vi "andor camera info.vi"(2 "error in":errorcluster) -> (0 "error out":errorcluster, 1 "Andor Camera Properties":T1)   [LabVIEW 2015]
uses:
  andor camera properties.ctl
  Program Files (x86)/BDS2006/ATMCD32D.DLL
panel:
  out "VS Speeds (us/row)":sgl[](array[numeric])
  out "Number of VS Speeds":i32
  out "Preamp Gain Settings":sgl[](array[numeric])
  out "Number of Preamp Gains":i32
  out "Pixel V (um)":sgl
  out "Pixel H (um)":sgl
  out "Pixel Frequencies (MHz)\n(for each channel)":sgl[][](array[numeric])
  out "Number of HS Speeds\n(for each Channel)":i32[](array[numeric])
  out "Number of AD Channels":i32
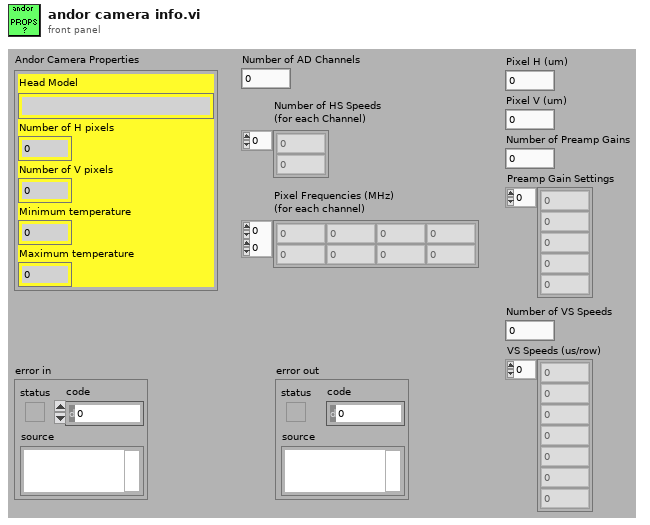
[diagram p1: front panel]
types:
  T1 = typedef "andor camera properties.ctl" = cluster{"Head Model":string, "Number of H pixels":i32, "Number of V pixels":i32, "Minimum temperature":i32, "Maximum temperature":i32}
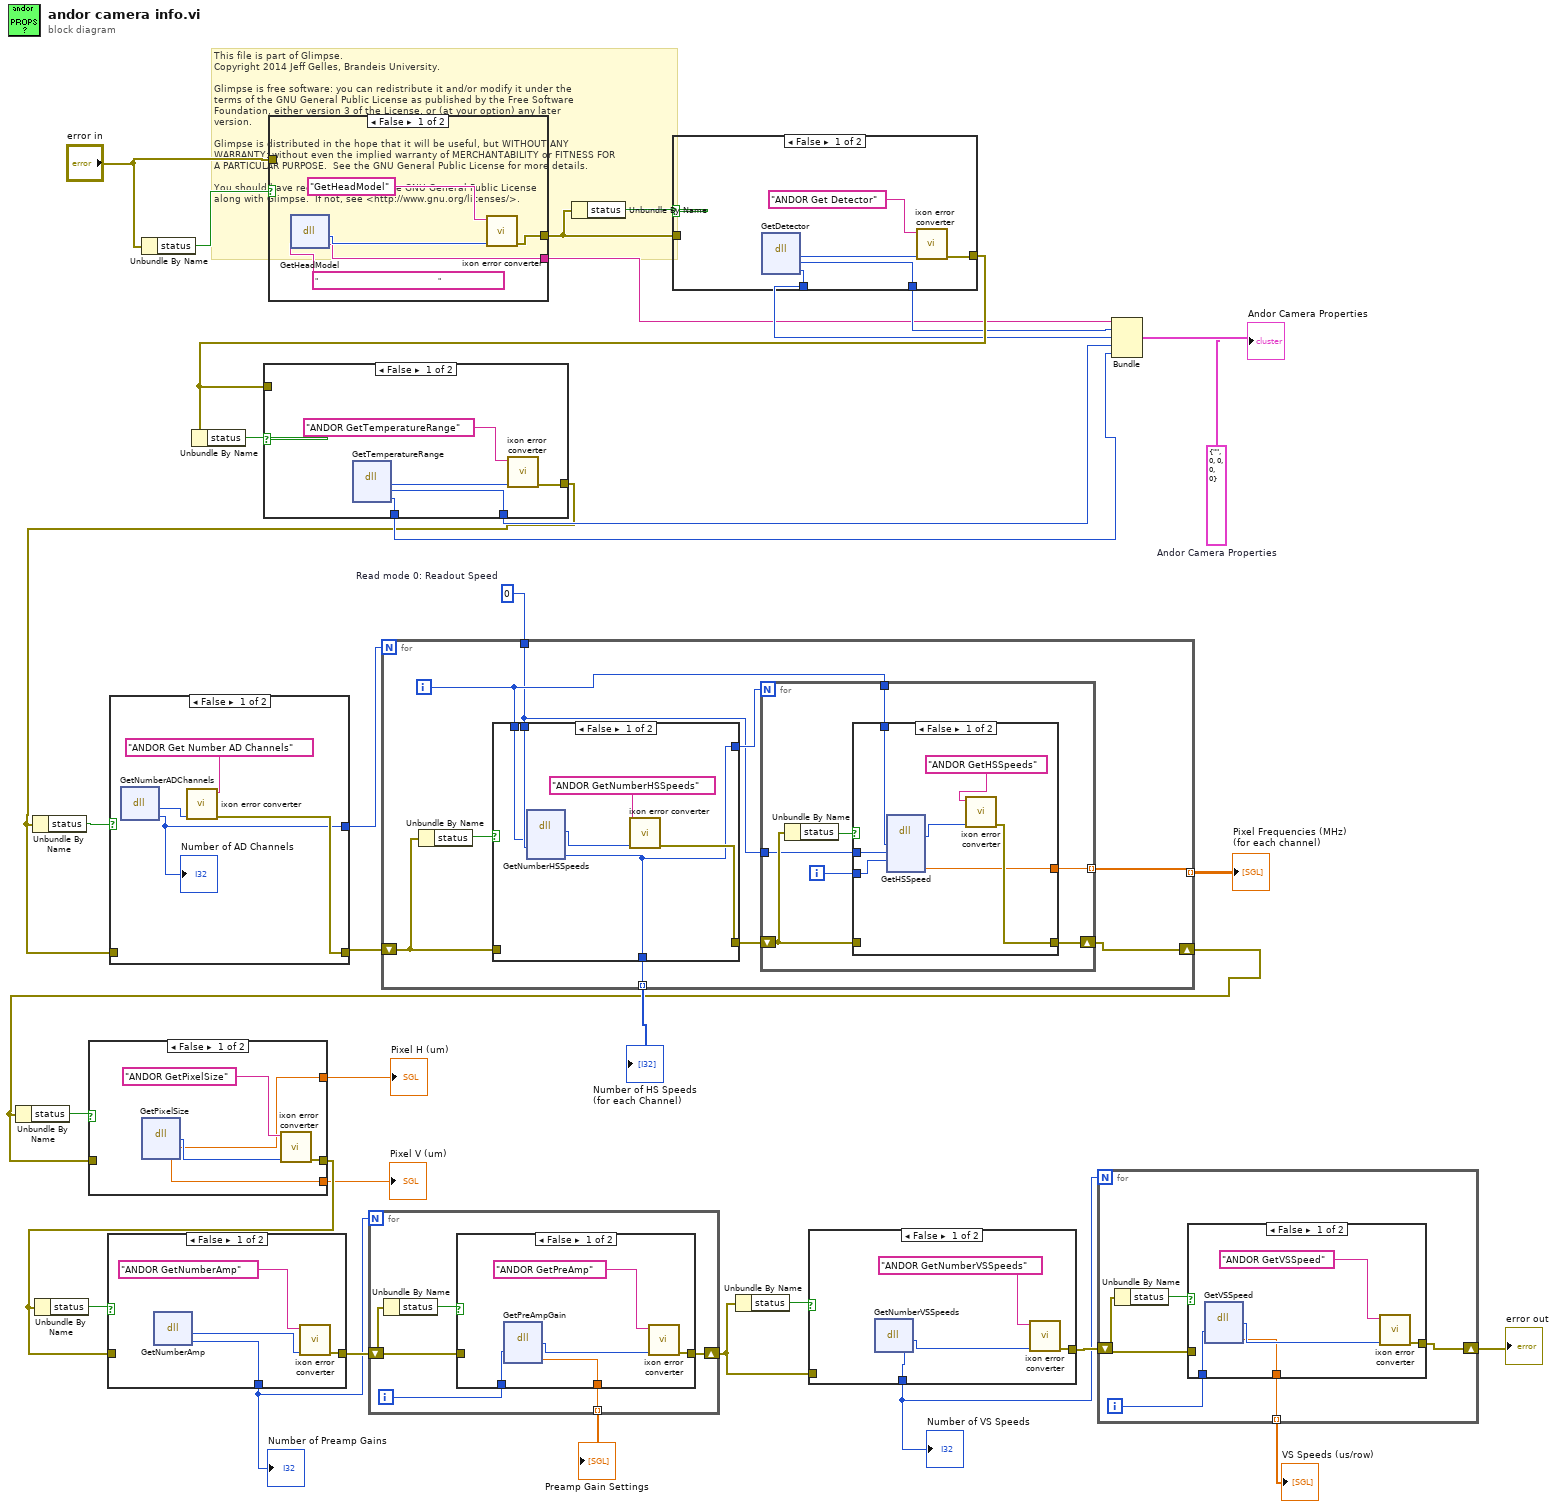
[diagram p0: block diagram]
diagram:
  w19 = 0  # Read mode 0: Readout Speed
  w27 = T1 {"Head Model"="", "Number of H pixels"=0, "Number of V pixels"=0, "Minimum temperature"=0, "Maximum temperature"=0}  # Andor Camera Properties
  # "This file is part of Glimpse. \nCopyright 2014 Jeff Gelles, Brandeis University.    \n\nGlimpse is free software: you can redistribute it and/or modify it under the \nterms of the GNU General Public License as published by the Free Software \nFoundation, either version 3 of the License, or (at your option) any later \nversion.\n\nGlimpse is distributed in the hope that it will be useful, but WITHOUT ANY \nWARRANTY; without even the implied warranty of MERCHANTABILITY or FITNESS FOR \nA PARTICULAR PURPOSE.  See the GNU General Public License for more details.\n\nYou should have received a copy of the GNU General Public License\nalong with Glimpse.  If not, see <http://www.gnu.org/licenses/>."
  n1 = Unbundle By Name("error in") -> ("status"=w24:bool)
  n2 = case shown="False" w24 {
    tunnel: [w38 w41] -> w26
    tunnel: "error in" -> [_ w41]
    tunnel: [w36 _] -> w28
    frame False {
      n3 = dll-call lib="C:/Program Files (x86)/BDS2006/Atmcd32d.dll" fn="GetHeadModel"("                                                            ") -> (w40:u32, w36:string)  [unwired: 3 in, 2 out]
      n4 = call "ixon error converter.vi"("Andor error code"=w40, "source"="GetHeadModel") -> ("error out"=w38:errorcluster)  [unwired: 5 out]
    }
    frame True {
    }
  }
  n5 = Unbundle By Name(w26) -> ("status"=w23:bool)
  n6 = case shown="False" w23 {
    tunnel: [w45 w47] -> w33
    tunnel: w26 -> [_ w47]
    tunnel: [w43 _] -> w29
    tunnel: [w42 _] -> w30
    frame False {
      n7 = dll-call lib="C:/Program Files (x86)/BDS2006/Atmcd32d.dll" fn="GetDetector" label="Get Detector"() -> (w44:u32, w42:i32, w43:i32)  [unwired: 3 in, 4 out]
      n8 = call "ixon error converter.vi"("Andor error code"=w44, "source"="ANDOR Get Detector") -> ("error out"=w45:errorcluster)  [unwired: 5 out]
    }
    frame True {
    }
  }
  n9 = Unbundle By Name(w33) -> ("status"=w32:bool)
  n10 = case shown="False" w32 {
    tunnel: [w51 w53] -> w22
    tunnel: [w49 _] -> w35
    tunnel: [w48 _] -> w34
    tunnel: w33 -> [_ w53]
    frame False {
      n11 = dll-call lib="C:/Program Files (x86)/BDS2006/Atmcd32d.dll" fn="GetTemperatureRange"() -> (w50:u32, w48:i32, w49:i32)  [unwired: 3 in, 4 out]
      n12 = call "ixon error converter.vi"("Andor error code"=w50, "source"="ANDOR GetTemperatureRange") -> ("error out"=w51:errorcluster)  [unwired: 5 out]
    }
    frame True {
    }
  }
  n13 = Unbundle By Name(w22) -> ("status"=w21:bool)
  n14 = case shown="False" w21 {
    tunnel: [w55 w58] -> w20
    tunnel: w22 -> [_ w58]
    tunnel: [w54 _] -> w1
    frame False {
      n15 = dll-call lib="C:/Program Files (x86)/BDS2006/Atmcd32d.dll" fn="GetNumberADChannels" label="Get Number AD Channels"() -> (w56:u32, w54:i32)  [unwired: 3 in, 3 out]
      "Number of AD Channels" <- w54
      n16 = call "ixon error converter.vi"("Andor error code"=w56, "source"="ANDOR Get Number AD Channels") -> ("error out"=w55:errorcluster)  [unwired: 5 out]
    }
    frame True {
    }
  }
  n17 = for {
    N: w1 -> [_]
    tunnel: [w66] -> w17 mode=indexing
    tunnel: w19 -> [w59]
    shift-right: [w61] -> w14
    shift-left: w20 -> [w64]
    tunnel: [w62] -> w18 mode=indexing
    i -> [w60]
    n18 = Unbundle By Name(w64) -> ("status"=w63:bool)
    n19 = case shown="False" w63 {
      tunnel: [w86 w89] -> w67
      tunnel: [w83 _] -> w65
      tunnel: w64 -> [_ w89]
      tunnel: w59 -> [w85 _]
      tunnel: w60 -> [w84 _]
      tunnel: [w83 _] -> w62
      frame False {
        n20 = dll-call lib="C:/Program Files (x86)/BDS2006/Atmcd32d.dll" fn="GetNumberHSSpeeds"(w84, w85) -> (w87:u32, w83:i32)  [unwired: 5 in, 3 out]
        n21 = call "ixon error converter.vi"("Andor error code"=w87, "source"="ANDOR GetNumberHSSpeeds") -> ("error out"=w86:errorcluster)  [unwired: 5 out]
      }
      frame True {
      }
    }
    n22 = for {
      N: w65 -> [_]
      shift-right: [w72] -> w61
      shift-left: w67 -> [w73]
      tunnel: [w71] -> w66 mode=indexing
      tunnel: w60 -> [w69]
      tunnel: w59 -> [w68]
      i -> [w70]
      n23 = Unbundle By Name(w73) -> ("status"=w74:bool)
      n24 = case shown="False" w74 {
        tunnel: w73 -> [_ w82]
        tunnel: [w79 w82] -> w72
        tunnel: [w78 _] -> w71
        tunnel: w70 -> [w77 _]
        tunnel: w69 -> [w76 _]
        tunnel: w68 -> [w75 _]
        frame False {
          n25 = dll-call lib="C:/Program Files (x86)/BDS2006/Atmcd32d.dll" fn="GetHSSpeed"(w76, w75, w77) -> (w80:u32, w78:sgl)  [unwired: 6 in, 3 out]
          n26 = call "ixon error converter.vi"("Andor error code"=w80, "source"="ANDOR GetHSSpeeds") -> ("error out"=w79:errorcluster)  [unwired: 5 out]
        }
        frame True {
        }
      }
    }
  }
  "Number of HS Speeds\n(for each Channel)" <- w18
  "Pixel Frequencies (MHz)\n(for each channel)" <- w17
  n27 = Unbundle By Name(w14) -> ("status"=w15:bool)
  n28 = case shown="False" w15 {
    tunnel: [w93 w95] -> w13
    tunnel: w14 -> [_ w95]
    tunnel: [w91 _] -> w11
    tunnel: [w90 _] -> w10
    frame False {
      n29 = dll-call lib="C:/Program Files (x86)/BDS2006/Atmcd32d.dll" fn="GetPixelSize"() -> (w92:u32, w90:sgl, w91:sgl)  [unwired: 3 in, 4 out]
      n30 = call "ixon error converter.vi"("Andor error code"=w92, "source"="ANDOR GetPixelSize") -> ("error out"=w93:errorcluster)  [unwired: 5 out]
    }
    frame True {
    }
  }
  "Pixel H (um)" <- w10
  "Pixel V (um)" <- w11
  n31 = Unbundle By Name(w13) -> ("status"=w16:bool)
  n32 = case shown="False" w16 {
    tunnel: [w98 w100] -> w12
    tunnel: w13 -> [_ w100]
    tunnel: [w97 _] -> w9
    frame False {
      n33 = dll-call lib="C:/Program Files (x86)/BDS2006/Atmcd32d.dll" fn="GetNumberAmp"() -> (w96:u32, w97:i32)  [unwired: 3 in, 3 out]
      n34 = call "ixon error converter.vi"("Andor error code"=w96, "source"="ANDOR GetNumberAmp") -> ("error out"=w98:errorcluster)  [unwired: 5 out]
    }
    frame True {
    }
  }
  "Number of Preamp Gains" <- w9
  n35 = for {
    N: w9 -> [_]
    tunnel: [w102] -> w8 mode=indexing
    shift-right: [w101] -> w7
    shift-left: w12 -> [w104]
    i -> [w103]
    n36 = Unbundle By Name(w104) -> ("status"=w105:bool)
    n37 = case shown="False" w105 {
      tunnel: [w109 w111] -> w101
      tunnel: w104 -> [_ w111]
      tunnel: w103 -> [w107 _]
      tunnel: [w106 _] -> w102
      frame False {
        n38 = dll-call lib="C:/Program Files (x86)/BDS2006/Atmcd32d.dll" fn="GetPreAmpGain" label="GetPreAmp"(w107) -> (w108:u32, w106:sgl)  [unwired: 4 in, 3 out]
        n39 = call "ixon error converter.vi"("Andor error code"=w108, "source"="ANDOR GetPreAmp") -> ("error out"=w109:errorcluster)  [unwired: 5 out]
      }
      frame True {
      }
    }
  }
  "Preamp Gain Settings" <- w8
  n40 = Unbundle By Name(w7) -> ("status"=w6:bool)
  n41 = case shown="False" w6 {
    tunnel: [w114 w116] -> w5
    tunnel: w7 -> [_ w116]
    tunnel: [w112 _] -> w4
    frame False {
      n42 = dll-call lib="C:/Program Files (x86)/BDS2006/Atmcd32d.dll" fn="GetNumberVSSpeeds"() -> (w113:u32, w112:i32)  [unwired: 3 in, 3 out]
      n43 = call "ixon error converter.vi"("Andor error code"=w113, "source"="ANDOR GetNumberVSSpeeds") -> ("error out"=w114:errorcluster)  [unwired: 5 out]
    }
    frame True {
    }
  }
  "Number of VS Speeds" <- w4
  n44 = for {
    N: w4 -> [_]
    shift-right: [w121] -> w2
    shift-left: w5 -> [w120]
    tunnel: [w118] -> w3 mode=indexing
    i -> [w119]
    n45 = Unbundle By Name(w120) -> ("status"=w117:bool)
    n46 = case shown="False" w117 {
      tunnel: [w125 w127] -> w121
      tunnel: w120 -> [_ w127]
      tunnel: w119 -> [w123 _]
      tunnel: [w122 _] -> w118
      frame False {
        n47 = dll-call lib="C:/Program Files (x86)/BDS2006/Atmcd32d.dll" fn="GetVSSpeed"(w123) -> (w124:u32, w122:sgl)  [unwired: 4 in, 3 out]
        n48 = call "ixon error converter.vi"("Andor error code"=w124, "source"="ANDOR GetVSSpeed") -> ("error out"=w125:errorcluster)  [unwired: 5 out]
      }
      frame True {
      }
    }
  }
  "error out" <- w2
  "VS Speeds (us/row)" <- w3
  n49 = Bundle(cluster=w27, "Head Model"=w28, "Number of H pixels"=w30, "Number of V pixels"=w29, "Minimum temperature"=w34, "Maximum temperature"=w35) -> (→"Andor Camera Properties":T1)
